vi "json Create.vi"(8 "error in (no error)":errorcluster, 10 "JSON String":string) -> (0 "error out":errorcluster, 3 "JSON Document out":refnum<class "JSON Document.lvclass">)   [LabVIEW 2015, in "JSON Document.lvclass"]
uses:
  JSON Document.lvclass
  JSON Document.lvclass/JSON Document.ctl
  rapidjson wrapper/rapidjson wrapper.lvlib
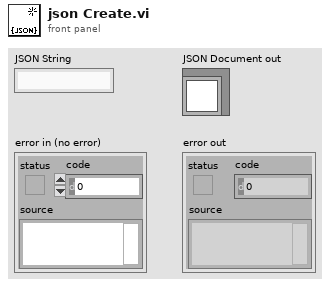
[diagram p1: front panel]
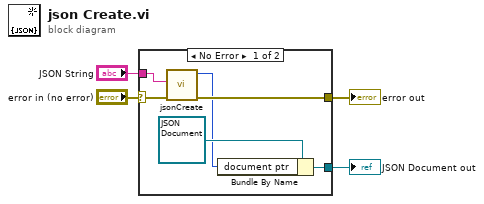
[diagram p0: block diagram]
diagram:
  n1 = case shown="No Error" "error in (no error)" {
    selector: "error in (no error)" -> [w10 w11]
    tunnel: [w9 w11] -> w3
    tunnel: "JSON String" -> [w8 _]
    tunnel: [w5 _] -> w1
    frame No Error {
      n2 = call "jsonCreate.vi"("error in (no error)"=w10, "json"=w8) -> ("error out"=w9:errorcluster, "return type"=w6:i64)  [unwired: 8 in]
      n3 = Bundle By Name(cluster=refnum<class "JSON Document.lvclass"> refnum ("JSON Document.lvclass"), "document ptr"=w6) -> (w5:refnum<class "JSON Document.lvclass">)
    }
    frame Error {
    }
  }
  "error out" <- w3
  "JSON Document out" <- w1
